vi "CheckLOT.vi"(8 "错误输入":errorcluster) -> (0 "错误输出":errorcluster, 3 "LOT":string)   [LabVIEW 2019]
panel:
  out "大小":i32[](array[numeric])
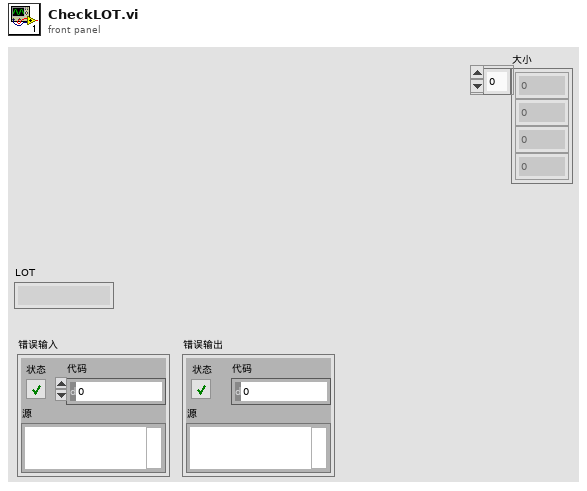
[diagram p1: front panel]
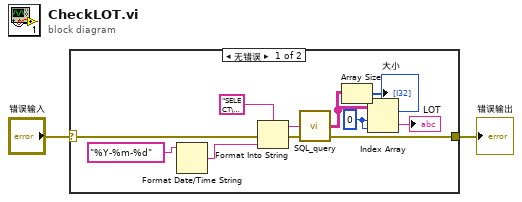
[diagram p0: block diagram]
diagram:
  n1 = case shown="无错误" "错误输入" {
    selector: "错误输入" -> [w7 w14]
    tunnel: [w5 w14] -> w1
    frame No Error {
      w9 = 0 ("索引 (行)")
      n2 = Format Date/Time String(time format string (%c)="%Y-%m-%d" ("时间格式字符串(%c)")) -> (date/time string=w11:string)  [unwired: 2 in]
      n3 = Format Into String(format string="SELECT\ndbo.[生产计划].[生产编号]\n\nFROM\ndbo.[生产计划]\nWHERE\ndbo.[生产计划].[日期] = '%s' AND\ndbo.[生产计划].[计划状态] = '已审核'", error in=w7, w11) -> (resulting string=w10:string, error out=w6:errorcluster)  [unwired: 1 in]
      n4 = call "SQL_query.vi"("error in (no error)"=w6, "SQL query"=w10) -> ("error out"=w5:errorcluster, "data"=w4:string[][])  [unwired: 1 in, 1 out]
      n5 = Array Size(array=w4) -> (size(s)=→"大小":i32[])
      n6 = Index Array(array=w4, index (row)=w9, index (col)=w9) -> (element=→"LOT":string)
    }
    frame Error {
    }
  }
  "错误输出" <- w1
